vi "CheckFutureColission.vi"(0 "object in":refnum<class "Events.lvclass">, 1 "RobotPos":dbl[](array[numeric]), 2 "Future Pos":dbl[](array[numeric]), 3 "Current Pos":dbl[](array[numeric]), 4 "DistanceForPossession":dbl, 5 "error in (no error)":errorcluster) -> (14 "object out":refnum<class "Events.lvclass">, 16 "touch":bool, 19 "error out":errorcluster)   [LabVIEW 2023, in "Events.lvclass"]
uses:
  Events.lvclass
  Utilities_class/Utilities.lvclass
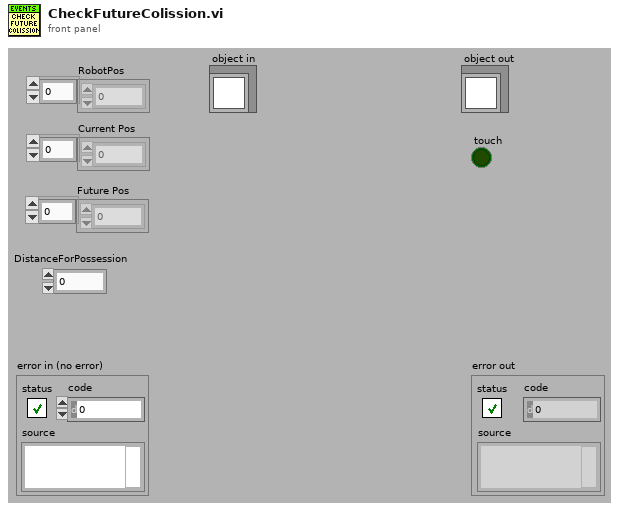
[diagram p1: front panel]
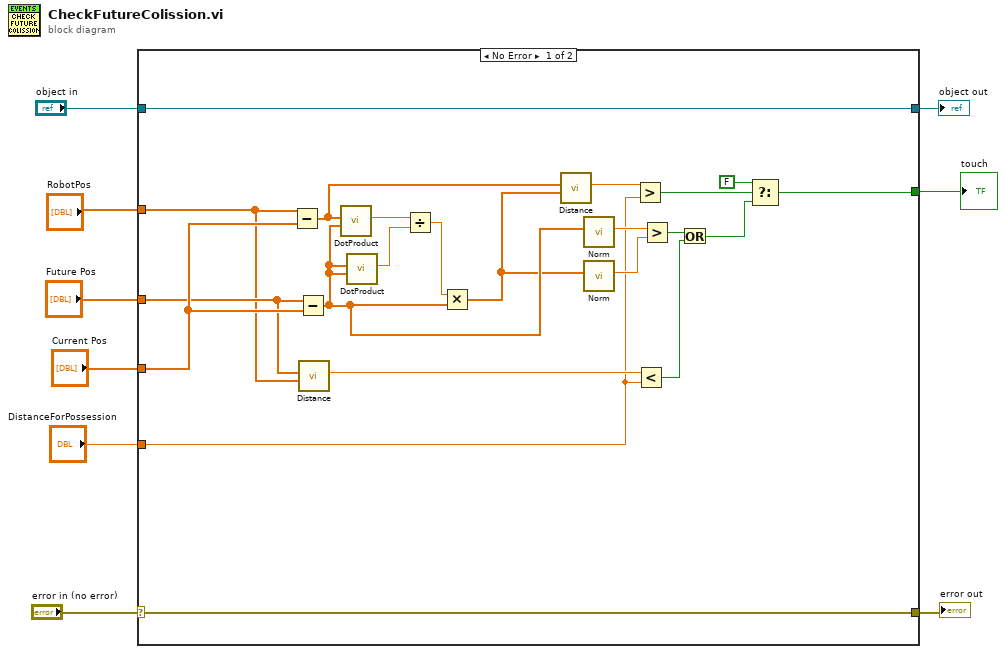
[diagram p0: block diagram]
diagram:
  n1 = case shown="No Error" "error in (no error)" {
    selector: "error in (no error)" -> [w30 w33]
    tunnel: [w30 w33] -> w8
    tunnel: [w31 w32] -> w6
    tunnel: "object in" -> [w31 w32]
    tunnel: "RobotPos" -> [w14 _]
    tunnel: "Current Pos" -> [w29 _]
    tunnel: "Future Pos" -> [w15 _]
    tunnel: "DistanceForPossession" -> [w12 _]
    tunnel: [w24 _] -> w1
    frame No Error {
      n2 = Subtract(x=w14, y=w29) -> (x-y=w18:dbl[])
      n3 = Subtract(x=w15, y=w29) -> (x-y=w23:dbl[])
      n4 = call "Distance.vi"("P1"=w14, "P2"=w15) -> ("Distance"=w13:dbl)  [unwired: 7 in, 2 out]
      n5 = call "DotProduct.vi"("Point2"=w23, "Point1"=w18) -> ("dot product"=w28:dbl)  [unwired: 7 in, 2 out]
      n6 = call "DotProduct.vi"("Point2"=w23, "Point1"=w23) -> ("dot product"=w27:dbl)  [unwired: 7 in, 2 out]
      n7 = Divide(x=w28, y=w27) -> (x/y=w26:dbl)
      n8 = Multiply(x=w26, y=w23) -> (x*y=w17:dbl[])
      n9 = call "Distance.vi"("P1"=w17, "P2"=w18) -> ("Distance"=w16:dbl)  [unwired: 7 in, 2 out]
      n10 = call "Norm.vi"("2D vector"=w23) -> ("Modulo"=w22:dbl)  [unwired: 8 in, 2 out]
      n11 = call "Norm.vi"("2D vector"=w17) -> ("Modulo"=w21:dbl)  [unwired: 8 in, 2 out]
      n12 = Greater?(x=w16, y=w12) -> (0:w25:bool)
      n13 = Less?(x=w13, y=w12) -> (x < y?=w11:bool)
      n14 = Greater?(x=w22, y=w21) -> (0:w20:bool)
      n15 = Or(x=w20, y=w11) -> (x .or. y?=w19:bool)
      n16 = Select(t=FALSE, s=w25, f=w19) -> (s? t:f=w24:bool)
    }
    frame Error {
    }
  }
  "error out" <- w8
  "object out" <- w6
  "touch" <- w1
